vi "sub_cDAQ_config.vi"(8 "error in":errorcluster caption="에러 입력") -> (0 "error out":errorcluster caption="에러 출력", 3 "task out":refnum<k21> caption="태스크 출력")   [LabVIEW 2016]
uses:
  <vilib>/DAQmx/configure/timing.llb/DAQmx Timing (Sample Clock).vi
  <vilib>/DAQmx/create/channels.llb/DAQmx Create Channel (AI-Strain-Strain Gage).vi
  <vilib>/DAQmx/create/channels.llb/DAQmx Create Channel (AI-Voltage-Basic).vi
  Global.vi
  <resource>/objmgr/daqmx.rc
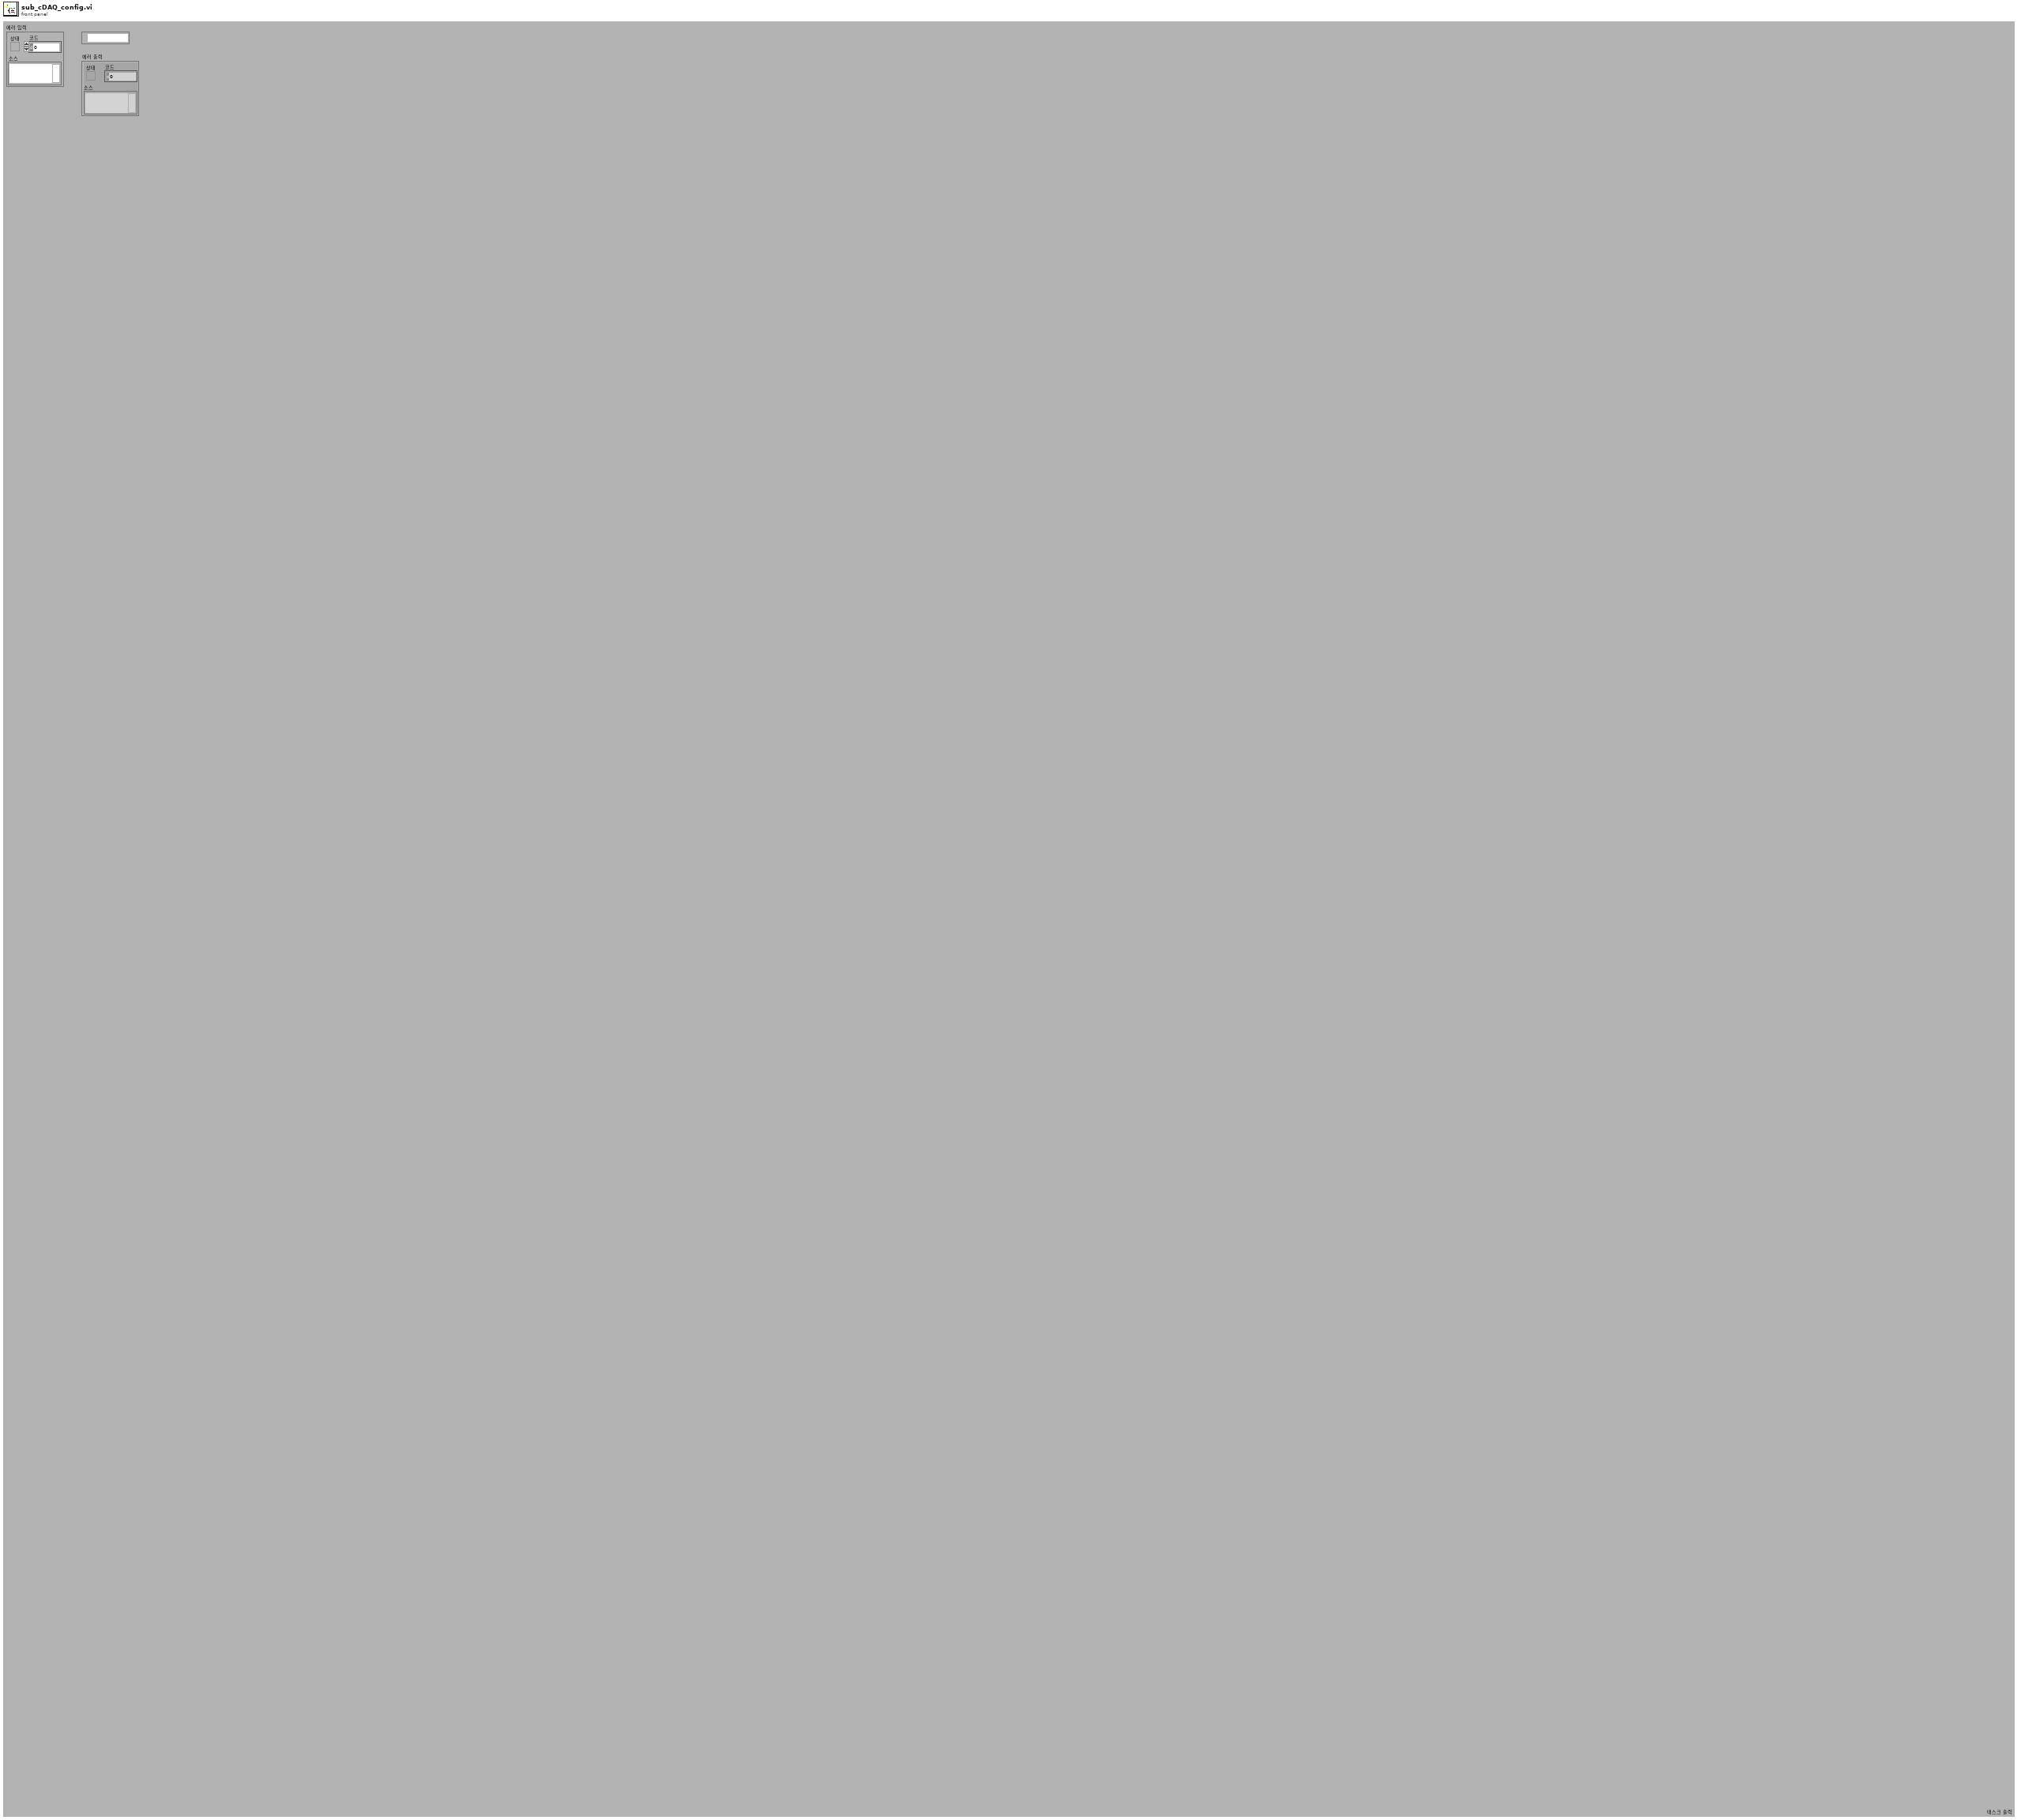
[diagram p1: front panel]
types:
  T1 = cluster{"strain configuration":i32, "lead resistance":dbl, "initial bridge voltage":dbl, "excitation source":i32, "excitation value":dbl}
  T2 = cluster{"gage factor":dbl, "nominal gage resistance":dbl, "poisson ratio":dbl}
  T3 = cluster{"sampling rate":dbl, "sample to read":dbl}
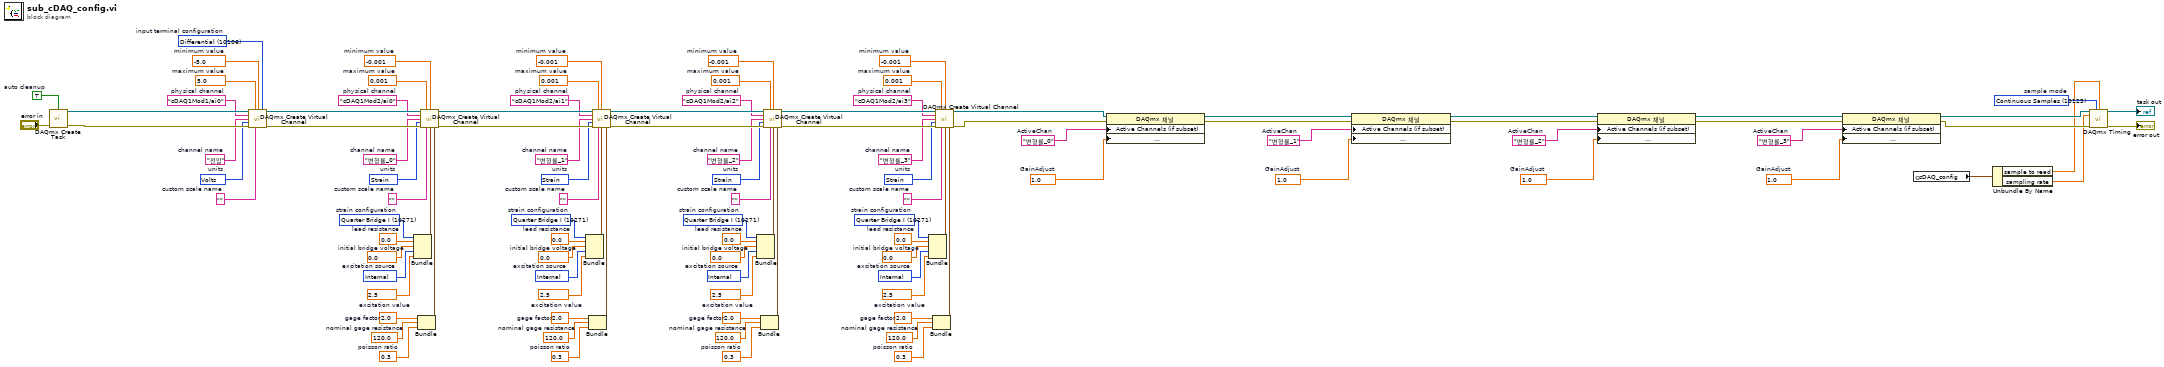
[diagram p0: block diagram]
diagram:
  w4 = 10123 items=["Finite Samples"=10178, "Continuous Samples"=10123, "Hardware Timed Single Point"=12522]  # sample mode
  w8 = 1.0  # GainAdjust
  w11 = "변형률_3"  # ActiveChan
  w12 = 1.0  # GainAdjust
  w15 = "변형률_2"  # ActiveChan
  w16 = 1.0  # GainAdjust
  w19 = "변형률_1"  # ActiveChan
  w20 = 1.0  # GainAdjust
  w23 = "변형률_0"  # ActiveChan
  w28 = 0.0  # lead resistance
  w31 = 0.3  # poisson ratio
  w27 = 0.0  # initial bridge voltage
  w32 = 120.0  # nominal gage resistance
  w30 = 2.0  # gage factor
  w25 = 2.5  # excitation value
  w26 = 10200 items=["Internal"=10200, "External"=10167, "None"=10230]  # excitation source
  w29 = 10271 items=["Full Bridge I"=10183, "Full Bridge II"=10184, "Full Bridge III"=10185, "Half Bridge I"=10188, "Half Bridge II"=10189, "Quarter Bridge I"=10271, "Quarter Bridge II"=10272]  # strain configuration
  w34 = 10299 items=["Strain"=10299, "From Custom Scale"=10065]  # units
  w35 = "변형률_3"  # channel name
  w37 = ""  # custom scale name
  w38 = -0.001  # minimum value
  w39 = 0.001  # maximum value
  w40 = "cDAQ1Mod2/ai3"  # physical channel
  w46 = 0.0  # lead resistance
  w49 = 0.3  # poisson ratio
  w45 = 0.0  # initial bridge voltage
  w50 = 120.0  # nominal gage resistance
  w48 = 2.0  # gage factor
  w43 = 2.5  # excitation value
  w44 = 10200 items=["Internal"=10200, "External"=10167, "None"=10230]  # excitation source
  w47 = 10271 items=["Full Bridge I"=10183, "Full Bridge II"=10184, "Full Bridge III"=10185, "Half Bridge I"=10188, "Half Bridge II"=10189, "Quarter Bridge I"=10271, "Quarter Bridge II"=10272]  # strain configuration
  w52 = 10299 items=["Strain"=10299, "From Custom Scale"=10065]  # units
  w53 = "변형률_2"  # channel name
  w55 = ""  # custom scale name
  w56 = -0.001  # minimum value
  w57 = 0.001  # maximum value
  w58 = "cDAQ1Mod2/ai2"  # physical channel
  w64 = 0.0  # lead resistance
  w67 = 0.3  # poisson ratio
  w63 = 0.0  # initial bridge voltage
  w68 = 120.0  # nominal gage resistance
  w66 = 2.0  # gage factor
  w61 = 2.5  # excitation value
  w62 = 10200 items=["Internal"=10200, "External"=10167, "None"=10230]  # excitation source
  w65 = 10271 items=["Full Bridge I"=10183, "Full Bridge II"=10184, "Full Bridge III"=10185, "Half Bridge I"=10188, "Half Bridge II"=10189, "Quarter Bridge I"=10271, "Quarter Bridge II"=10272]  # strain configuration
  w70 = 10299 items=["Strain"=10299, "From Custom Scale"=10065]  # units
  w71 = "변형률_1"  # channel name
  w73 = ""  # custom scale name
  w74 = -0.001  # minimum value
  w75 = 0.001  # maximum value
  w76 = "cDAQ1Mod2/ai1"  # physical channel
  w82 = 0.0  # lead resistance
  w85 = 0.3  # poisson ratio
  w81 = 0.0  # initial bridge voltage
  w86 = 120.0  # nominal gage resistance
  w84 = 2.0  # gage factor
  w79 = 2.5  # excitation value
  w80 = 10200 items=["Internal"=10200, "External"=10167, "None"=10230]  # excitation source
  w83 = 10271 items=["Full Bridge I"=10183, "Full Bridge II"=10184, "Full Bridge III"=10185, "Half Bridge I"=10188, "Half Bridge II"=10189, "Quarter Bridge I"=10271, "Quarter Bridge II"=10272]  # strain configuration
  w88 = 10299 items=["Strain"=10299, "From Custom Scale"=10065]  # units
  w89 = "변형률_0"  # channel name
  w91 = ""  # custom scale name
  w92 = -0.001  # minimum value
  w93 = 0.001  # maximum value
  w94 = "cDAQ1Mod2/ai0"  # physical channel
  w96 = 10106 items=["default"=-1, "RSE"=10083, "NRSE"=10078, "Differential"=10106, "Pseudodifferential"=12529]  # input terminal configuration
  w97 = 10348 items=["Volts"=10348, "From Custom Scale"=10065]  # units
  w98 = "전압"  # channel name
  w100 = ""  # custom scale name
  w101 = -5.0  # minimum value
  w102 = 5.0  # maximum value
  w103 = "cDAQ1Mod1/ai0"  # physical channel
  w105 = TRUE  # auto cleanup
  n1 = call <vilib>:"DAQmx Create Task.vi"("auto cleanup"=w105, "error in"="error in") -> ("task out"=w104:refnum<k21>, "error out"=w106:errorcluster)  [unwired: 12 in]
  n2 = call-poly <vilib>:"DAQmx Create Virtual Channel.vi"("task in"=w104, "maximum value"=w102, "minimum value"=w101, "input terminal configuration"=w96, "physical channels"=w103, "name to assign"=w98, "units"=w97, "error in"=w106, "custom scale name"=w100) -> ("task out"=w95:refnum<k21>, "error out"=w99:errorcluster)  [unwired: 5 in]
  n3 = Bundle("strain configuration"=w83, "lead resistance"=w82, "initial bridge voltage"=w81, "excitation source"=w80, "excitation value"=w79) -> (w78:T1)  [unwired: 1 in]
  n4 = Bundle("gage factor"=w84, "nominal gage resistance"=w86, "poisson ratio"=w85) -> (w87:T2)  [unwired: 1 in]
  n5 = call-poly <vilib>:"DAQmx Create Virtual Channel.vi"("task in"=w95, "maximum value"=w93, "minimum value"=w92, "physical channels"=w94, "name to assign"=w89, "units"=w88, "error in"=w99, "custom scale name"=w91, "bridge information"=w78, "strain gage information"=w87) -> ("task out"=w77:refnum<k21>, "error out"=w90:errorcluster)  [unwired: 4 in]
  n6 = Bundle("strain configuration"=w65, "lead resistance"=w64, "initial bridge voltage"=w63, "excitation source"=w62, "excitation value"=w61) -> (w60:T1)  [unwired: 1 in]
  n7 = Bundle("gage factor"=w66, "nominal gage resistance"=w68, "poisson ratio"=w67) -> (w69:T2)  [unwired: 1 in]
  n8 = call-poly <vilib>:"DAQmx Create Virtual Channel.vi"("task in"=w77, "maximum value"=w75, "minimum value"=w74, "physical channels"=w76, "name to assign"=w71, "units"=w70, "error in"=w90, "custom scale name"=w73, "bridge information"=w60, "strain gage information"=w69) -> ("task out"=w59:refnum<k21>, "error out"=w72:errorcluster)  [unwired: 4 in]
  n9 = Bundle("strain configuration"=w47, "lead resistance"=w46, "initial bridge voltage"=w45, "excitation source"=w44, "excitation value"=w43) -> (w42:T1)  [unwired: 1 in]
  n10 = Bundle("gage factor"=w48, "nominal gage resistance"=w50, "poisson ratio"=w49) -> (w51:T2)  [unwired: 1 in]
  n11 = call-poly <vilib>:"DAQmx Create Virtual Channel.vi"("task in"=w59, "maximum value"=w57, "minimum value"=w56, "physical channels"=w58, "name to assign"=w53, "units"=w52, "error in"=w72, "custom scale name"=w55, "bridge information"=w42, "strain gage information"=w51) -> ("task out"=w41:refnum<k21>, "error out"=w54:errorcluster)  [unwired: 4 in]
  n12 = Bundle("strain configuration"=w29, "lead resistance"=w28, "initial bridge voltage"=w27, "excitation source"=w26, "excitation value"=w25) -> (w24:T1)  [unwired: 1 in]
  n13 = Bundle("gage factor"=w30, "nominal gage resistance"=w32, "poisson ratio"=w31) -> (w33:T2)  [unwired: 1 in]
  n14 = call-poly <vilib>:"DAQmx Create Virtual Channel.vi"("task in"=w41, "maximum value"=w39, "minimum value"=w38, "physical channels"=w40, "name to assign"=w35, "units"=w34, "error in"=w54, "custom scale name"=w37, "bridge information"=w24, "strain gage information"=w33) -> ("task out"=w22:refnum<k21>, "error out"=w36:errorcluster)  [unwired: 4 in]
  n15 = property class="DAQmx 채널"(reference=w22, error in=w36, "Active Channels (if subset)"=w23, "Analog Input:General Properties:Signal Conditioning:Bridge:Shunt Cal:Gain Adjustment"=w20) -> (reference out=w18:refnum<k21>, error out=w21:errorcluster)
  n16 = property class="DAQmx 채널"(reference=w18, error in=w21, "Active Channels (if subset)"=w19, "Analog Input:General Properties:Signal Conditioning:Bridge:Shunt Cal:Gain Adjustment"=w16) -> (reference out=w14:refnum<k21>, error out=w17:errorcluster)
  n17 = property class="DAQmx 채널"(reference=w14, error in=w17, "Active Channels (if subset)"=w15, "Analog Input:General Properties:Signal Conditioning:Bridge:Shunt Cal:Gain Adjustment"=w12) -> (reference out=w10:refnum<k21>, error out=w13:errorcluster)
  n18 = property class="DAQmx 채널"(reference=w10, error in=w13, "Active Channels (if subset)"=w11, "Analog Input:General Properties:Signal Conditioning:Bridge:Shunt Cal:Gain Adjustment"=w8) -> (reference out=w5:refnum<k21>, error out=w9:errorcluster)
  n19 = global read "Global.vi" "cDAQ_config"() -> (w3:T3)
  n20 = Unbundle By Name(w3) -> ("sample to read"=w1:dbl, "sampling rate"=w2:dbl)
  n21 = call-poly <vilib>:"DAQmx Timing.vi"("task/channels in"=w5, "sample mode"=w4, "samples per channel"=w1, "rate"=w2, "error in"=w9) -> ("task out"=→"task out":refnum<k21>, "error out"=→"error out":errorcluster)  [unwired: 9 in]
